vi "scan_string.vi"() -> ()   [LabVIEW 2021]
panel:
  out "error out":errorcluster
  out "resulting string":string
  out "inserted string":string
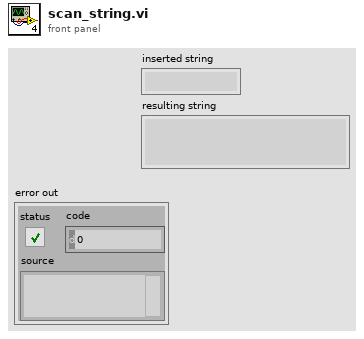
[diagram p1: front panel]
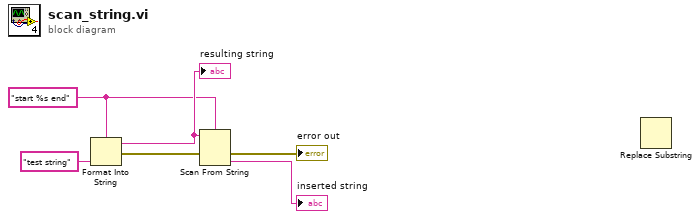
[diagram p0: block diagram]
diagram:
  w1 = "start %s end" ("format string")
  n1 = Format Into String "Format Into String"(format string=w1, "test string" ("input 1")) -> (resulting string=w4:string, error out=w6:errorcluster)  [unwired: 2 in]
  "resulting string" <- w4
  n2 = Scan From String "Scan From String"(format string=w1, input string=w4, error in=w6) -> (error out=→"error out":errorcluster, output 1=→"inserted string":string)  [unwired: 2 in, 2 out]
  n3 = Replace Substring() -> ()  [unwired: 4 in, 2 out]
